vi "General setup bundler-String.vi"(7 "Section":string, 8 "error in (no error)":errorcluster, 10 "String":T2, 11 "Setup.ini ref":T1) -> (0 "error out":errorcluster, 3 "Setup.ini ref":T1)   [LabVIEW 2020]
uses:
  <vilib>/Utility/config.llb/Config Data RefNum.ctl
  Typedefs/Ini file interface (String).ctl
  Global Variables/General Globals.vi
  <vilib>/Utility/config.llb/NI_LVConfig.lvlib
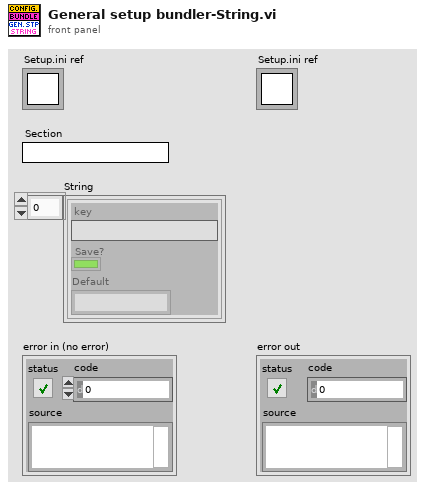
[diagram p1: front panel]
types:
  T1 = typedef "NI_LVConfig.lvlib/Config Data RefNum.ctl" = refnum<k1>
  T2 = typedef "Ini file interface (String).ctl" = cluster{"key":string, "Save?":bool, "Default":string}[]
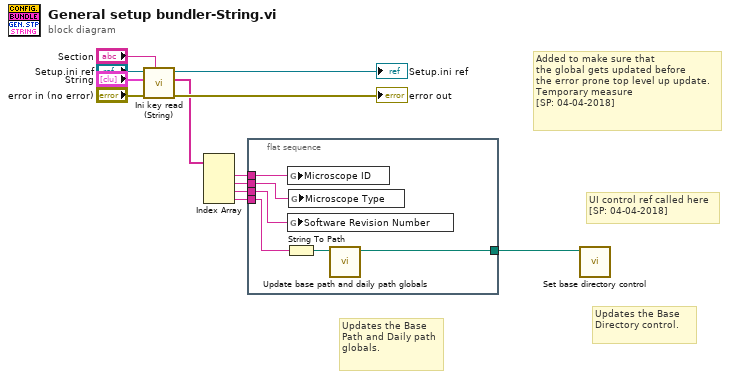
[diagram p0: block diagram]
diagram:
  # "Added to make sure that\nthe global gets updated before \nthe error prone top level up update.Temporary measure\n[SP: 04-04-2018]"
  # "UI control ref called here\n[SP: 04-04-2018]"
  # "Updates the Base Path and Daily path globals."
  # "Updates the Base Directory control."
  n1 = call "Ini key read (String).vi"("Section name"="Section", "error in (no error)"="error in (no error)", "Keys setup"="String", "Ini file ref in"="Setup.ini ref") -> ("error out"=→"error out":errorcluster, "Value read/used"=w9:string[], "Ini file ref"=→"Setup.ini ref":T1)  [unwired: 5 in]
  n2 = Index Array(array=w9) -> (element #1=w4:string, element #2=w3:string, element #3=w2:string, element #4=w1:string)  [unwired: 4 in]
  n3 = flat-sequence {
    tunnel: [w17] -> w5
    tunnel: w4 -> [w16]
    tunnel: w3 -> [w15]
    tunnel: w2 -> [w14]
    tunnel: w1 -> [w13]
    frame #0 {
      n4 = String To Path(string=w13) -> (path=w18:path)
      n5 = global write "General Globals.vi" "Microscope ID"(w16) -> ()
      n6 = global write "General Globals.vi" "Software Revision Number"(w14) -> ()
      n7 = global write "General Globals.vi" "Microscope Type"(w15) -> ()
      n8 = call "Update base path and daily path globals.vi"("Base Directory"=w18) -> ("Base Directory (dupl)"=w17:path)  [unwired: 9 in, 1 out]
    }
  }
  n9 = call "Set base directory control.vi"("Base path"=w5) -> ()  [unwired: 10 in, 1 out]
